vi "9870 Interface DMA (FPGA).vi"() -> ()   [LabVIEW 2014]
uses:
  <vilib>/LabVIEW Targets/FPGA/cRIO/shared/nicrio_ModuleControls/nicrio_cRIO-9871_BaudRateEnum.ctl
  <vilib>/LabVIEW Targets/FPGA/cRIO/shared/nicrio_ModuleControls/nicrio_cRIO-9871_DataBitsEnum.ctl
  <vilib>/LabVIEW Targets/FPGA/cRIO/shared/nicrio_ModuleControls/nicrio_cRIO-9871_ParityEnum.ctl
  <vilib>/LabVIEW Targets/FPGA/cRIO/shared/nicrio_ModuleControls/nicrio_cRIO-9871_StopBitsEnum.ctl
  <vilib>/LabVIEW Targets/FPGA/cRIO/shared/nicrio_ModuleControls/nicrio_cRIO-9871_FlowControlEnum.ctl
  <vilib>/rvi/Emulation/niFpgaGetClockAttributes.vi
  <vilib>/rvi/Emulation/niFpgaSctlEmulationGetInTimedLoop.vi
  <vilib>/rvi/Emulation/niFpgaEmulationReportErrorSimple.vi
  <vilib>/rvi/Emulation/niFpgaProcessEmulError.vi
  <vilib>/rvi/interface/RandomDataEmulation/niFpgaRandomDataHandleErrors.vi
  <vilib>/rvi/eio/common/nirviEmuTemplateMethod_errors.vi
  <vilib>/rvi/Emulation/niFpgaCriticalErrorInLSC.vi
  <vilib>/rvi/eio/common/nirviEmuTemplatePropertySet_errors.vi
  <vilib>/rvi/DataTransferAndStorage/Container/XNode/niFpgaContainer.xnode
  <vilib>/rvi/interface/RandomDataEmulation/nirviRandomDataFpgaReadWriteTemplate.vi
  <vilib>/eio/EIOMethodNode/EIOMethodNode.xnode
  <vilib>/eio/EIOPropertyNode/EIOPropertyNode.xnode
  <vilib>/rvi/eio/common/nirviEmuTemplatePropertyGet_errors.vi
  <vilib>/rvi/eio/common/nirviEmuTemplatePropertyGet_noerrors.vi
  <vilib>/rvi/eio/common/nirviEmuTemplatePropertySet_noerrors.vi
panel:
  in  "Write Data (FPGA2)":bool
  in  "Bytes to Send 2":i32
  in  "Port To Write (FPGA2)":enum8{"0", "1", "2", "3", "4"}(ring)
  out "error out 4b":errorcluster
  in  "Port 8":T6={"Baud Rate"=enum."9600 bps", "Data Bits"=enum."8", "Parity"=enum."None", "Stop Bits"=enum."1", "Flow Control"=enum."None"}
  in  "Port 7":T6={"Baud Rate"=enum."9600 bps", "Data Bits"=enum."8", "Parity"=enum."None", "Stop Bits"=enum."1", "Flow Control"=enum."None"}
  in  "Port 6":T6={"Baud Rate"=enum."9600 bps", "Data Bits"=enum."8", "Parity"=enum."None", "Stop Bits"=enum."1", "Flow Control"=enum."None"}
  in  "Port 5":T6={"Baud Rate"=enum."9600 bps", "Data Bits"=enum."8", "Parity"=enum."None", "Stop Bits"=enum."1", "Flow Control"=enum."None"}
  out "error out 5":errorcluster
  out "error out 6":errorcluster
  out "error out 7":errorcluster
  out "error out 8":errorcluster
  out "Error Out":errorcluster
  out "error out 4":errorcluster
  out "error out 3":errorcluster
  out "error out 2":errorcluster
  in  "Write Data (FPGA)":bool
  in  "Port To Write (FPGA)":enum8{"0", "1", "2", "3", "4"}(ring)
  in  "Port 1":T6={"Baud Rate"=enum."9600 bps", "Data Bits"=enum."8", "Parity"=enum."None", "Stop Bits"=enum."1", "Flow Control"=enum."None"}
  in  "Port 3":T6={"Baud Rate"=enum."9600 bps", "Data Bits"=enum."8", "Parity"=enum."None", "Stop Bits"=enum."1", "Flow Control"=enum."None"}
  in  "Port 4":T6={"Baud Rate"=enum."9600 bps", "Data Bits"=enum."8", "Parity"=enum."None", "Stop Bits"=enum."1", "Flow Control"=enum."None"}
  in  "Port 2":T6={"Baud Rate"=enum."9600 bps", "Data Bits"=enum."8", "Parity"=enum."None", "Stop Bits"=enum."1", "Flow Control"=enum."None"}
  in  "Bytes to Send":i32
  in  "Timeout (ms)":i32=1
  in  "Update Config":bool
  out "error out 1":errorcluster
  # "Port Read Timeout"
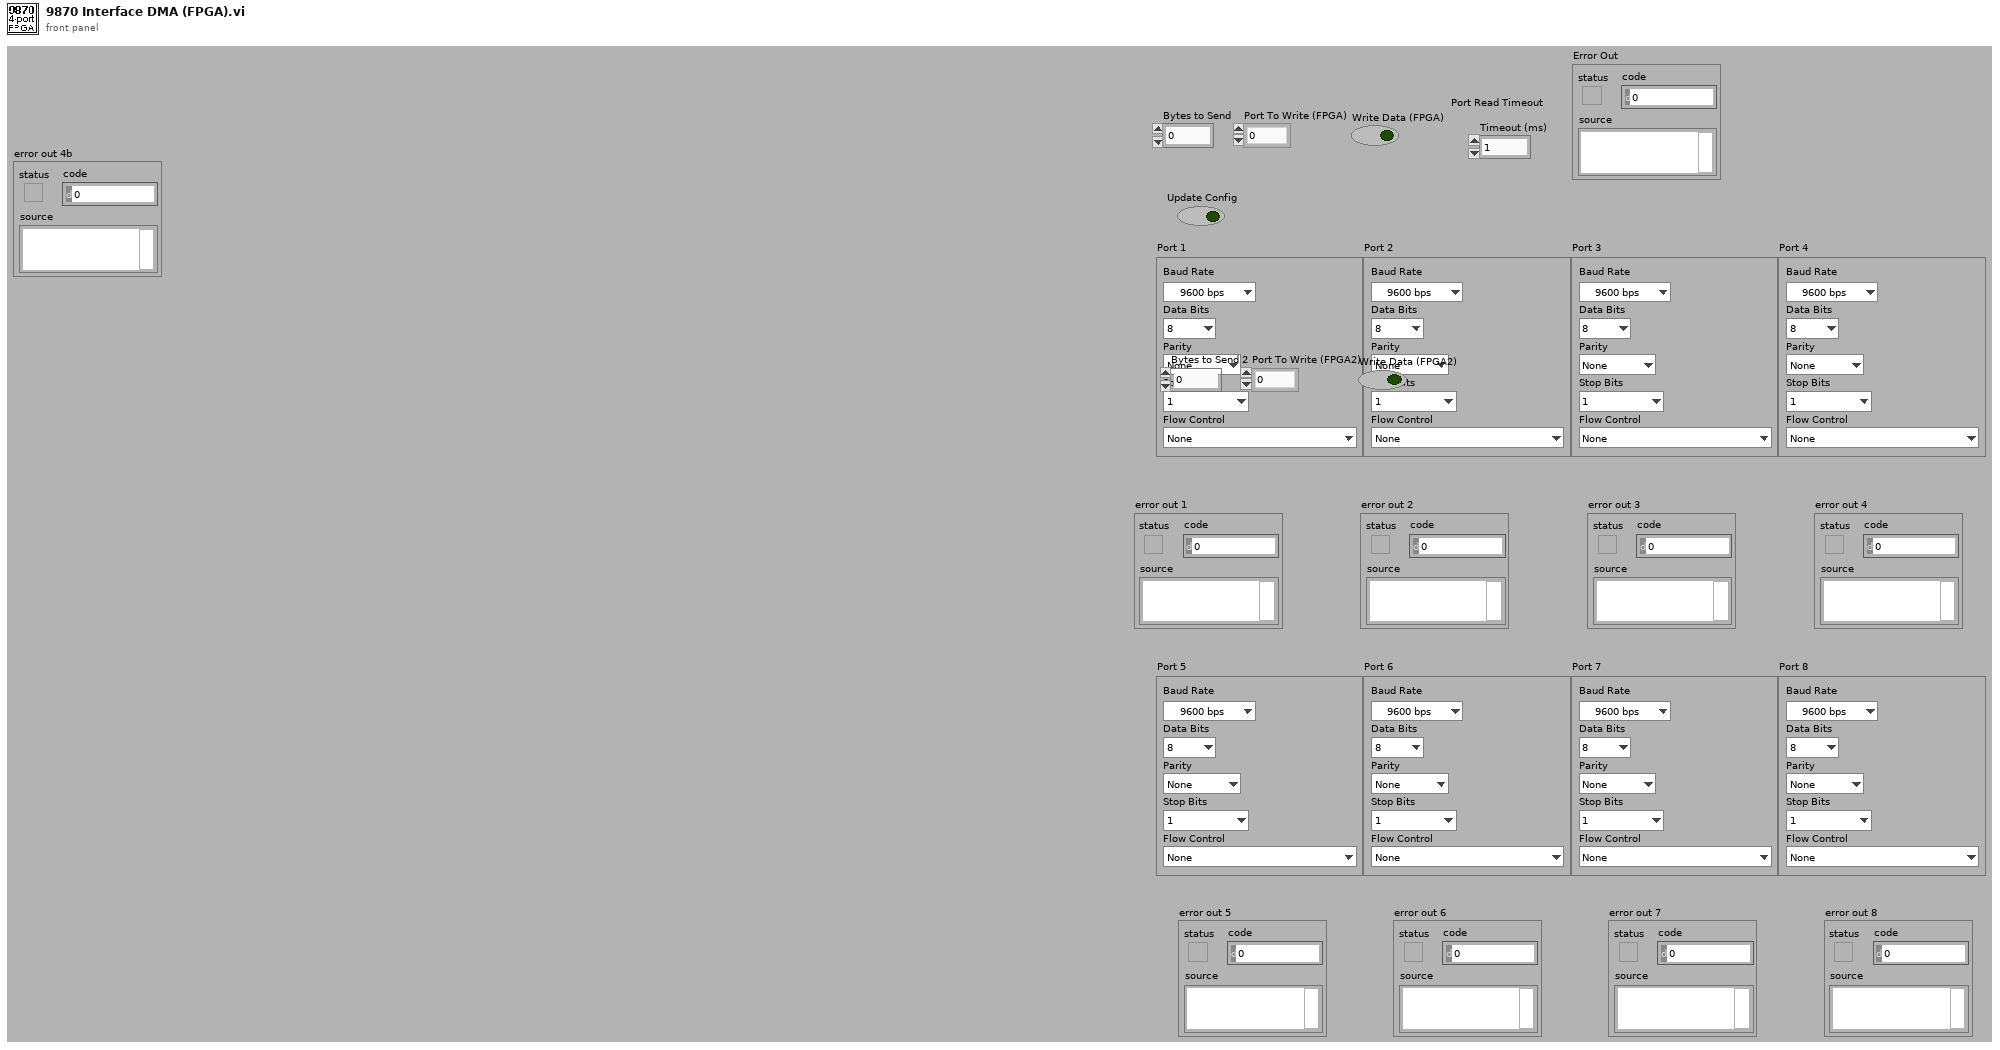
[diagram p1: front panel]
types:
  T1 = typedef "nicrio_cRIO-9871_BaudRateEnum.ctl" = enum16{"75 bps", "110 bps", "134 bps", "150 bps", "300 bps", "600 bps", "1200 bps", "1800 bps", "2400 bps", "4800 bps", "7200 bps", "9600 bps", "14.4 kbps", "19.2 kbps", "28.8 kbps", "38.4 kbps", "57.6 kbps", "115.2 kbps", "230.4 kbps", "460.8 kbps", "921.6 kbps"}
  T2 = typedef "nicrio_cRIO-9871_DataBitsEnum.ctl" = enum8{"5", "6", "7", "8"}
  T3 = typedef "nicrio_cRIO-9871_ParityEnum.ctl" = enum8{"None", "Odd", "Even", "Mark", "Space"}
  T4 = typedef "nicrio_cRIO-9871_StopBitsEnum.ctl" = enum8{"1", "1.5", "2"}
  T5 = typedef "nicrio_cRIO-9871_FlowControlEnum.ctl" = enum8{"None", "Software (XON / XOFF)", "Hardware (RTS / CTS)"}
  T6 = cluster{"Baud Rate":T1, "Data Bits":T2, "Parity":T3, "Stop Bits":T4, "Flow Control":T5}
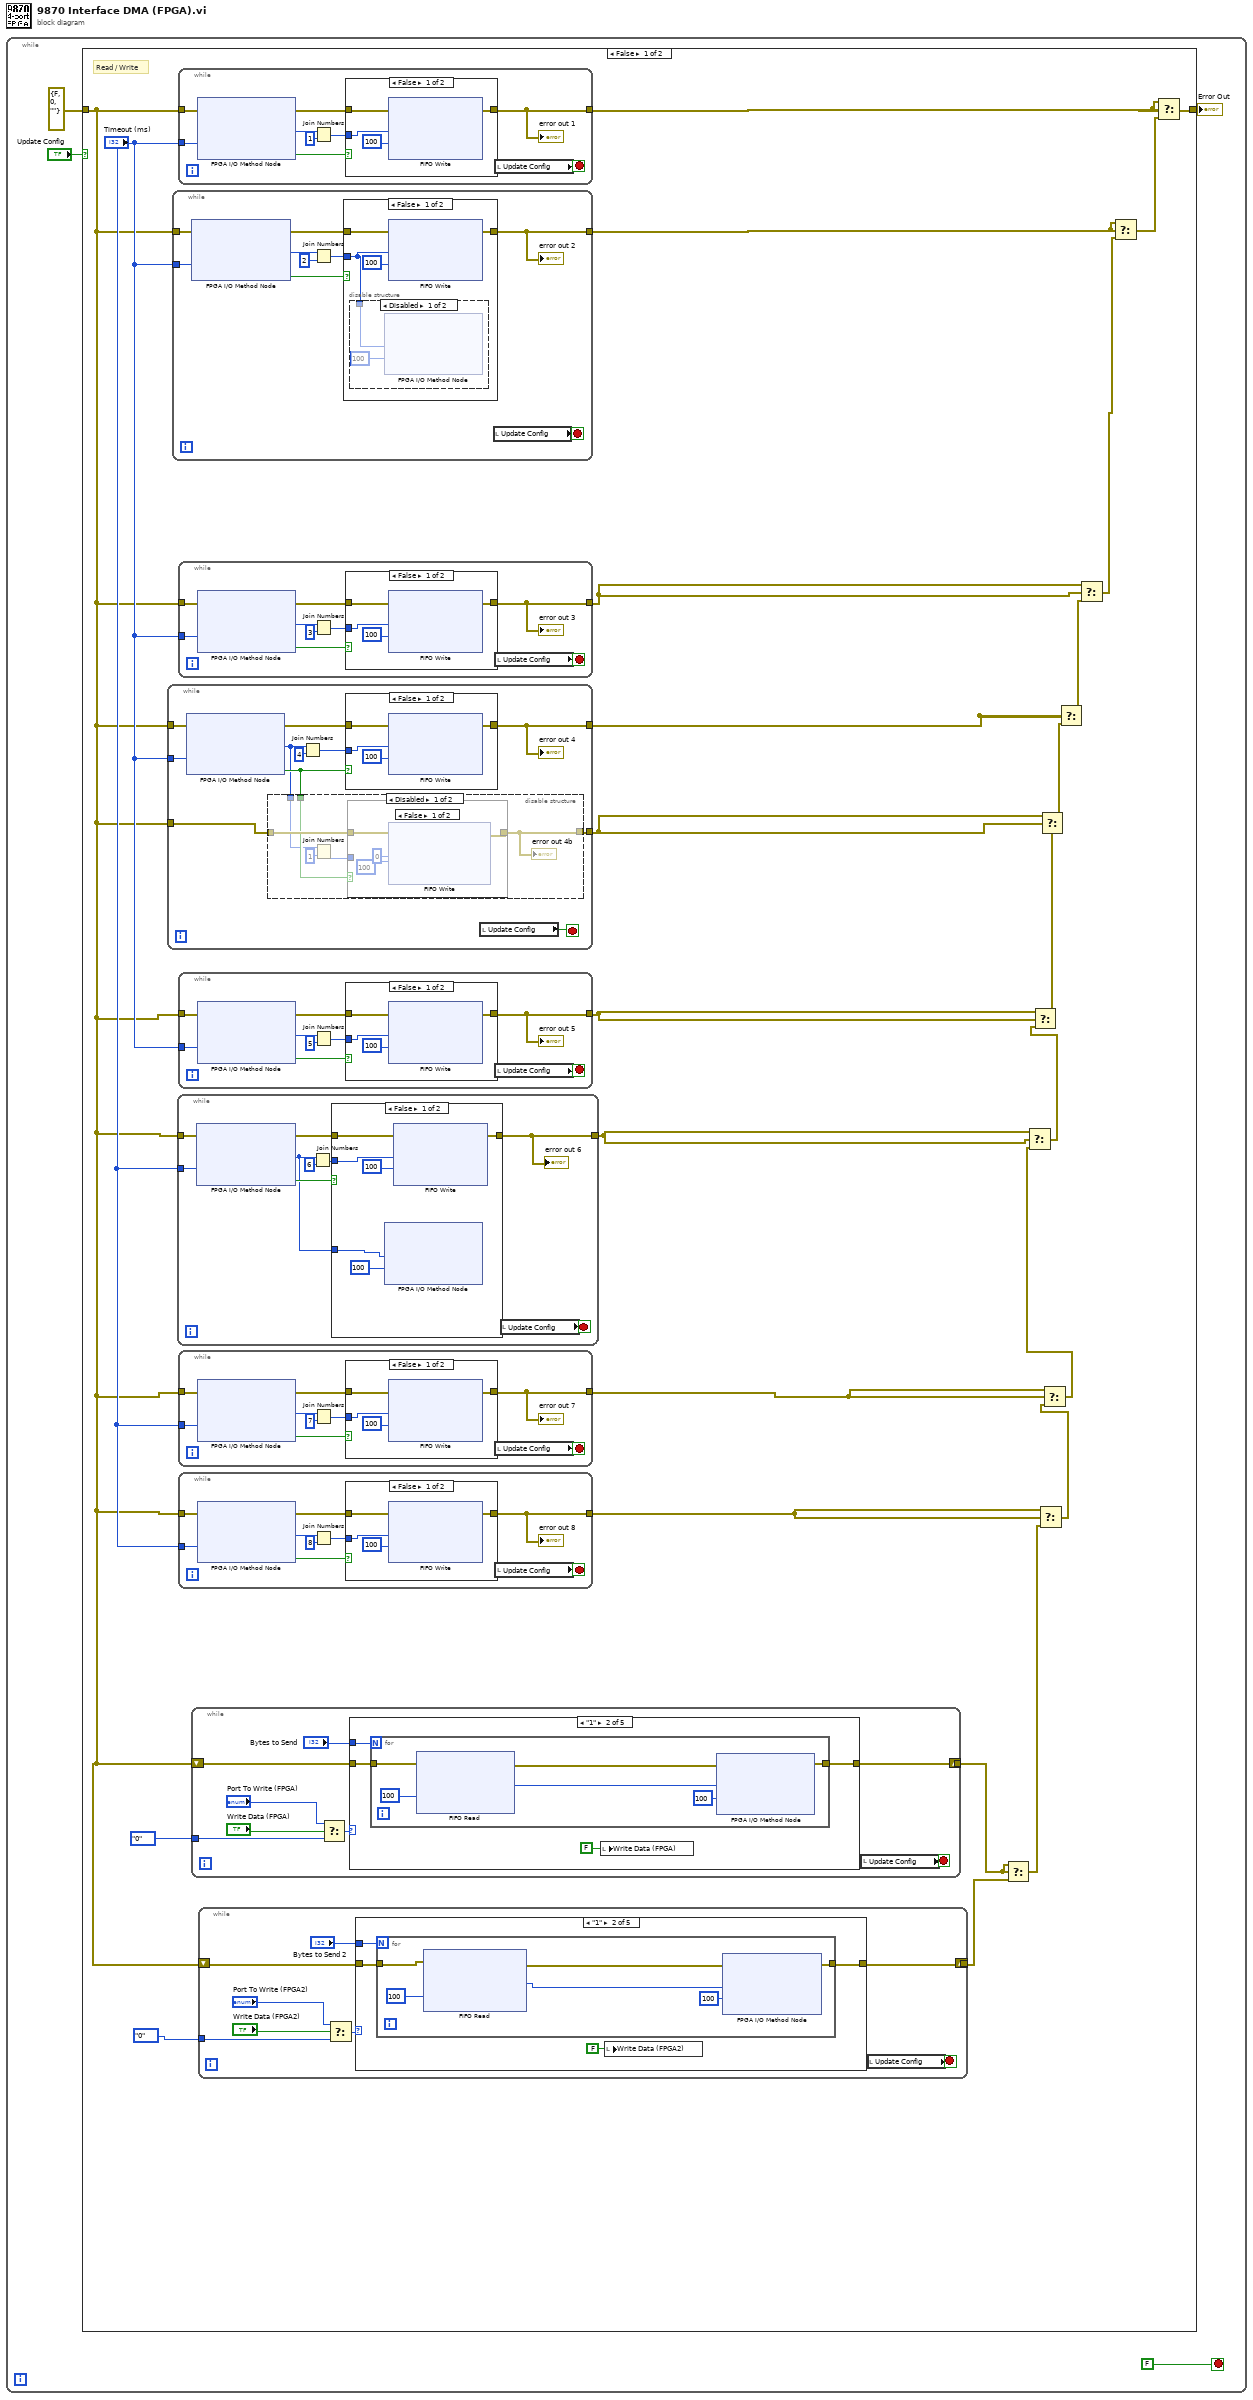
[diagram p0: block diagram]
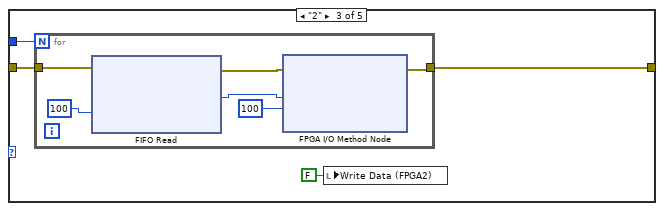
[diagram p3: hidden frame]
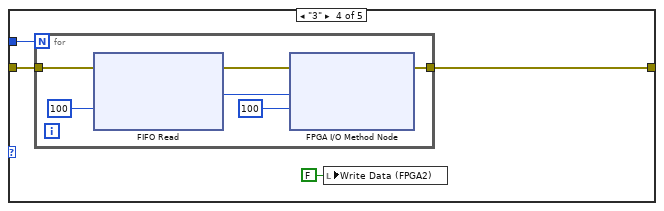
[diagram p4: hidden frame]
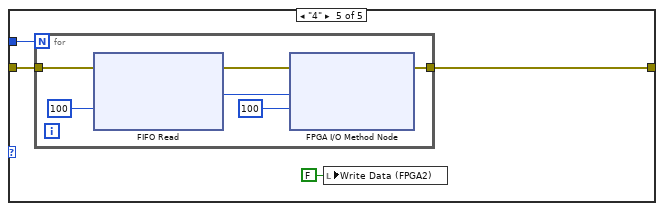
[diagram p5: hidden frame]
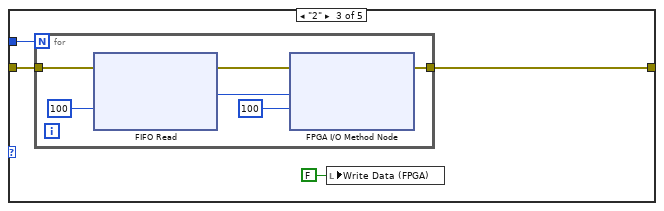
[diagram p17: hidden frame]
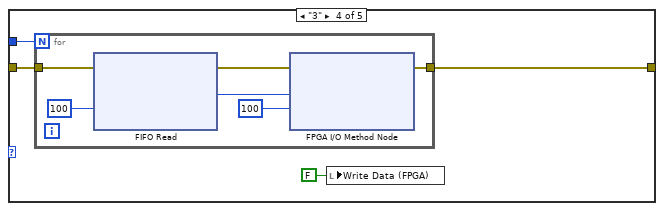
[diagram p18: hidden frame]
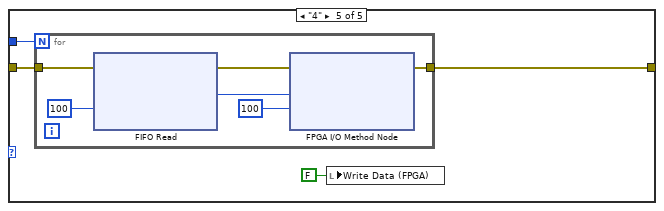
[diagram p19: hidden frame]
diagram:
  n1 = while {
    stop <- FALSE ("Boolean") stop-if-true
    n2 = case shown="False" "Update Config" {
      tunnel: [w23 w257] -> w1
      tunnel: errorcluster {"status"=FALSE, "code"=0, "source"=""} ("error out") -> [w9 w298]
      frame False {
        # "Read / Write"
        n3 = while {
          tunnel: "Timeout (ms)" -> [w144]
          tunnel: w9 -> [w147]
          tunnel: [w141] -> w22
          tunnel: w9 -> [w140]
          tunnel: [w137] -> w12
          stop <- w142 stop-if-true
          n4 = xnode "FPGA I/O Method Node"("error in"=w147, "Timeout (ms)"=w144) -> ("error out"=w143:errorcluster, "Data"=w138:u8, "Timed Out"=w139:bool)  [unwired: 1 in, 1 out]
          n5 = disable-structure shown="Disabled" {
            disable-tunnel: w140 -> [w153 _]
            disable-tunnel: w139 -> [w152 _]
            disable-tunnel: w138 -> [w151 _]
            disable-tunnel: [w150 _] -> w137
            frame Disabled {
              n6 = Join Numbers(hi=w151, lo=u8 1) -> ((hi.lo)=w148:u16)
              n7 = case shown="False" w152 {
                tunnel: w148 -> [_ _]
                tunnel: w153 -> [w157 w158]
                tunnel: [w156 w158] -> w150
                frame False {
                  n8 = xnode ("FIFO Write")("Element"=i16 0, "Timeout"=100, "error in (no error)"=w157) -> ("error out"=w156:errorcluster)  [unwired: 1 in, 2 out]
                }
                frame True {
                }
              }
              "error out 4b" <- w150
            }
            frame Enabled {
            }
          }
          n9 = Join Numbers(hi=w138, lo=u8 4) -> ((hi.lo)=w145:u16)
          n10 = case shown="False" w139 {
            tunnel: w145 -> [w161 _]
            tunnel: w143 -> [w160 w163]
            tunnel: [w159 w163] -> w141
            frame False {
              n11 = xnode ("FIFO Write")("Element"=w161, "Timeout"=100, "error in (no error)"=w160) -> ("error out"=w159:errorcluster)  [unwired: 1 in, 2 out]
            }
            frame True {
            }
          }
          "error out 4" <- w141
          n12 = local read "Update Config"() -> (w142:bool)
        }
        n13 = while {
          tunnel: "Timeout (ms)" -> [w182]
          tunnel: w9 -> [w186]
          tunnel: [w179] -> w28
          stop <- w180 stop-if-true
          n14 = xnode "FPGA I/O Method Node"("error in"=w186, "Timeout (ms)"=w182) -> ("error out"=w181:errorcluster, "Data"=w178:u8, "Timed Out"=w185:bool)  [unwired: 1 in, 1 out]
          n15 = Join Numbers(hi=w178, lo=u8 2) -> ((hi.lo)=w183:u16)
          n16 = case shown="False" w185 {
            tunnel: w183 -> [w187 _]
            tunnel: w181 -> [w189 w193]
            tunnel: [w188 w193] -> w179
            frame False {
              n17 = disable-structure shown="Disabled" {
                disable-tunnel: w187 -> [w191 _]
                frame Disabled {
                  n18 = xnode "FPGA I/O Method Node"("Data"=w191, "Timeout (ms)"=100 ("Timeout")) -> ()  [unwired: 2 in, 3 out]
                }
                frame Enabled {
                }
              }
              n19 = xnode ("FIFO Write")("Element"=w187, "Timeout"=100, "error in (no error)"=w189) -> ("error out"=w188:errorcluster)  [unwired: 1 in, 2 out]
            }
            frame True {
            }
          }
          "error out 2" <- w179
          n20 = local read "Update Config"() -> (w180:bool)
        }
        n21 = while {
          tunnel: "Timeout (ms)" -> [w111]
          tunnel: w9 -> [w115]
          tunnel: [w108] -> w15
          stop <- w109 stop-if-true
          n22 = xnode "FPGA I/O Method Node"("error in"=w115, "Timeout (ms)"=w111) -> ("error out"=w110:errorcluster, "Data"=w107:u8, "Timed Out"=w114:bool)  [unwired: 1 in, 1 out]
          n23 = Join Numbers(hi=w107, lo=u8 6) -> ((hi.lo)=w112:u16)
          n24 = case shown="False" w114 {
            tunnel: w112 -> [w120 _]
            tunnel: w110 -> [w119 w122]
            tunnel: [w118 w122] -> w108
            tunnel: w107 -> [w116 _]
            frame False {
              n25 = xnode "FPGA I/O Method Node"("Data"=w116, "Timeout (ms)"=100 ("Timeout")) -> ()  [unwired: 2 in, 3 out]
              n26 = xnode ("FIFO Write")("Element"=w120, "Timeout"=100, "error in (no error)"=w119) -> ("error out"=w118:errorcluster)  [unwired: 1 in, 2 out]
            }
            frame True {
            }
          }
          "error out 6" <- w108
          n27 = local read "Update Config"() -> (w109:bool)
        }
        n28 = while {
          tunnel: "Timeout (ms)" -> [w246]
          tunnel: w9 -> [w251]
          tunnel: [w243] -> w27
          stop <- w244 stop-if-true
          n29 = xnode "FPGA I/O Method Node"("error in"=w251, "Timeout (ms)"=w246) -> ("error out"=w245:errorcluster, "Data"=w249:u8, "Timed Out"=w250:bool)  [unwired: 1 in, 1 out]
          n30 = Join Numbers(hi=w249, lo=u8 1) -> ((hi.lo)=w247:u16)
          n31 = case shown="False" w250 {
            tunnel: w247 -> [w254 _]
            tunnel: w245 -> [w253 w256]
            tunnel: [w252 w256] -> w243
            frame False {
              n32 = xnode ("FIFO Write")("Element"=w254, "Timeout"=100, "error in (no error)"=w253) -> ("error out"=w252:errorcluster)  [unwired: 1 in, 2 out]
            }
            frame True {
            }
          }
          "error out 1" <- w243
          n33 = local read "Update Config"() -> (w244:bool)
        }
        n34 = while {
          tunnel: "Timeout (ms)" -> [w167]
          tunnel: w9 -> [w172]
          tunnel: [w164] -> w26
          stop <- w165 stop-if-true
          n35 = xnode "FPGA I/O Method Node"("error in"=w172, "Timeout (ms)"=w167) -> ("error out"=w166:errorcluster, "Data"=w170:u8, "Timed Out"=w171:bool)  [unwired: 1 in, 1 out]
          n36 = Join Numbers(hi=w170, lo=u8 3) -> ((hi.lo)=w168:u16)
          n37 = case shown="False" w171 {
            tunnel: w168 -> [w175 _]
            tunnel: w166 -> [w174 w177]
            tunnel: [w173 w177] -> w164
            frame False {
              n38 = xnode ("FIFO Write")("Element"=w175, "Timeout"=100, "error in (no error)"=w174) -> ("error out"=w173:errorcluster)  [unwired: 1 in, 2 out]
            }
            frame True {
            }
          }
          "error out 3" <- w164
          n39 = local read "Update Config"() -> (w165:bool)
        }
        n40 = while {
          tunnel: "Timeout (ms)" -> [w126]
          tunnel: w9 -> [w131]
          tunnel: [w123] -> w16
          stop <- w124 stop-if-true
          n41 = xnode "FPGA I/O Method Node"("error in"=w131, "Timeout (ms)"=w126) -> ("error out"=w125:errorcluster, "Data"=w129:u8, "Timed Out"=w130:bool)  [unwired: 1 in, 1 out]
          n42 = Join Numbers(hi=w129, lo=u8 5) -> ((hi.lo)=w127:u16)
          n43 = case shown="False" w130 {
            tunnel: w127 -> [w134 _]
            tunnel: w125 -> [w133 w136]
            tunnel: [w132 w136] -> w123
            frame False {
              n44 = xnode ("FIFO Write")("Element"=w134, "Timeout"=100, "error in (no error)"=w133) -> ("error out"=w132:errorcluster)  [unwired: 1 in, 2 out]
            }
            frame True {
            }
          }
          "error out 5" <- w123
          n45 = local read "Update Config"() -> (w124:bool)
        }
        n46 = while {
          tunnel: "Timeout (ms)" -> [w96]
          tunnel: w9 -> [w101]
          tunnel: [w93] -> w14
          stop <- w94 stop-if-true
          n47 = xnode "FPGA I/O Method Node"("error in"=w101, "Timeout (ms)"=w96) -> ("error out"=w95:errorcluster, "Data"=w99:u8, "Timed Out"=w100:bool)  [unwired: 1 in, 1 out]
          n48 = Join Numbers(hi=w99, lo=u8 7) -> ((hi.lo)=w97:u16)
          n49 = case shown="False" w100 {
            tunnel: w97 -> [w104 _]
            tunnel: w95 -> [w103 w106]
            tunnel: [w102 w106] -> w93
            frame False {
              n50 = xnode ("FIFO Write")("Element"=w104, "Timeout"=100, "error in (no error)"=w103) -> ("error out"=w102:errorcluster)  [unwired: 1 in, 2 out]
            }
            frame True {
            }
          }
          "error out 7" <- w93
          n51 = local read "Update Config"() -> (w94:bool)
        }
        n52 = while {
          tunnel: "Timeout (ms)" -> [w82]
          tunnel: w9 -> [w87]
          tunnel: [w79] -> w13
          stop <- w80 stop-if-true
          n53 = xnode "FPGA I/O Method Node"("error in"=w87, "Timeout (ms)"=w82) -> ("error out"=w81:errorcluster, "Data"=w85:u8, "Timed Out"=w86:bool)  [unwired: 1 in, 1 out]
          n54 = Join Numbers(hi=w85, lo=u8 8) -> ((hi.lo)=w83:u16)
          n55 = case shown="False" w86 {
            tunnel: w83 -> [w90 _]
            tunnel: w81 -> [w89 w92]
            tunnel: [w88 w92] -> w79
            frame False {
              n56 = xnode ("FIFO Write")("Element"=w90, "Timeout"=100, "error in (no error)"=w89) -> ("error out"=w88:errorcluster)  [unwired: 1 in, 2 out]
            }
            frame True {
            }
          }
          "error out 8" <- w79
          n57 = local read "Update Config"() -> (w80:bool)
        }
        n58 = while {
          shift-right: [w198] -> _
          shift-left: w9 -> [w201]
          tunnel: enum8{"0", "1", "2", "3", "4"}."0" ("Port To Write (FPGA) 2") -> [w196]
          tunnel: [w198] -> w6
          stop <- w200 stop-if-true
          n59 = Select(t="Port To Write (FPGA)", s="Write Data (FPGA)", f=w196) -> (s? t:f=w195:enum8{"0", "1", "2", "3", "4"})
          n60 = case shown="\"1\"" w195 {
            tunnel: w201 -> [w202 w206 w216 w226 w236]
            tunnel: "Bytes to Send" -> [_ w205 w215 w225 w235]
            tunnel: [w202 w204 w214 w224 w234] -> w198
            frame "0", Default {
            }
            frame "1" {
              n61 = for {
                N: w205 -> [_]
                tunnel: w206 -> [w212]
                tunnel: [w208] -> w204
                n62 = xnode ("FIFO Read")("Timeout"=100 ("Timeout (ms)"), "error in (no error)"=w212) -> ("Element"=w207:u8, "error out"=w211:errorcluster)  [unwired: 1 in, 2 out]
                n63 = xnode "FPGA I/O Method Node"("error in"=w211, "Data"=w207, "Timeout (ms)"=100) -> ("error out"=w208:errorcluster)  [unwired: 1 in, 2 out]
              }
              n64 = local write "Write Data (FPGA)"(FALSE ("Write Data (FPGA)")) -> ()
            }
            frame "2" {
              n65 = for {
                N: w215 -> [_]
                tunnel: w216 -> [w221]
                tunnel: [w217] -> w214
                n66 = xnode ("FIFO Read")("Timeout"=100 ("Timeout (ms)"), "error in (no error)"=w221) -> ("Element"=w222:u8, "error out"=w220:errorcluster)  [unwired: 1 in, 2 out]
                n67 = xnode "FPGA I/O Method Node"("error in"=w220, "Data"=w222, "Timeout (ms)"=100) -> ("error out"=w217:errorcluster)  [unwired: 1 in, 2 out]
              }
              n68 = local write "Write Data (FPGA)"(FALSE ("Write Data (FPGA)")) -> ()
            }
            frame "3" {
              n69 = for {
                N: w225 -> [_]
                tunnel: w226 -> [w231]
                tunnel: [w227] -> w224
                n70 = xnode ("FIFO Read")("Timeout"=100 ("Timeout (ms)"), "error in (no error)"=w231) -> ("Element"=w232:u8, "error out"=w230:errorcluster)  [unwired: 1 in, 2 out]
                n71 = xnode "FPGA I/O Method Node"("error in"=w230, "Data"=w232, "Timeout (ms)"=100) -> ("error out"=w227:errorcluster)  [unwired: 1 in, 2 out]
              }
              n72 = local write "Write Data (FPGA)"(FALSE ("Write Data (FPGA)")) -> ()
            }
            frame "4" {
              n73 = for {
                N: w235 -> [_]
                tunnel: w236 -> [w241]
                tunnel: [w237] -> w234
                n74 = xnode ("FIFO Read")("Timeout"=100 ("Timeout (ms)"), "error in (no error)"=w241) -> ("Element"=w242:u8, "error out"=w240:errorcluster)  [unwired: 1 in, 2 out]
                n75 = xnode "FPGA I/O Method Node"("error in"=w240, "Data"=w242, "Timeout (ms)"=100) -> ("error out"=w237:errorcluster)  [unwired: 1 in, 2 out]
              }
              n76 = local write "Write Data (FPGA)"(FALSE ("Write Data (FPGA)")) -> ()
            }
          }
          n77 = local read "Update Config"() -> (w200:bool)
        }
        n78 = while {
          shift-right: [w34] -> w7
          shift-left: w9 -> [w37]
          tunnel: enum8{"0", "1", "2", "3", "4"}."0" ("Port To Write (FPGA) 2") -> [w32]
          tunnel: [w34] -> _
          stop <- w36 stop-if-true
          n79 = Select(t="Port To Write (FPGA2)", s="Write Data (FPGA2)", f=w32) -> (s? t:f=w31:enum8{"0", "1", "2", "3", "4"})
          n80 = case shown="\"1\"" w31 {
            tunnel: w37 -> [w38 w42 w52 w62 w72]
            tunnel: "Bytes to Send 2" -> [_ w41 w51 w61 w71]
            tunnel: [w38 w40 w50 w60 w70] -> w34
            frame "0", Default {
            }
            frame "1" {
              n81 = for {
                N: w41 -> [_]
                tunnel: w42 -> [w48]
                tunnel: [w45] -> w40
                n82 = xnode ("FIFO Read")("Timeout"=100 ("Timeout (ms)"), "error in (no error)"=w48) -> ("Element"=w43:i16, "error out"=w47:errorcluster)  [unwired: 1 in, 2 out]
                n83 = xnode "FPGA I/O Method Node"("error in"=w47, "Data"=w43, "Timeout (ms)"=100) -> ("error out"=w45:errorcluster)  [unwired: 1 in, 2 out]
              }
              n84 = local write "Write Data (FPGA2)"(FALSE ("Write Data (FPGA)")) -> ()
            }
            frame "2" {
              n85 = for {
                N: w51 -> [_]
                tunnel: w52 -> [w58]
                tunnel: [w53] -> w50
                n86 = xnode ("FIFO Read")("Timeout"=100 ("Timeout (ms)"), "error in (no error)"=w58) -> ("Element"=w56:i16, "error out"=w54:errorcluster)  [unwired: 1 in, 2 out]
                n87 = xnode "FPGA I/O Method Node"("error in"=w54, "Data"=w56, "Timeout (ms)"=100) -> ("error out"=w53:errorcluster)  [unwired: 1 in, 2 out]
              }
              n88 = local write "Write Data (FPGA2)"(FALSE ("Write Data (FPGA)")) -> ()
            }
            frame "3" {
              n89 = for {
                N: w61 -> [_]
                tunnel: w62 -> [w67]
                tunnel: [w63] -> w60
                n90 = xnode ("FIFO Read")("Timeout"=100 ("Timeout (ms)"), "error in (no error)"=w67) -> ("Element"=w68:i16, "error out"=w66:errorcluster)  [unwired: 1 in, 2 out]
                n91 = xnode "FPGA I/O Method Node"("error in"=w66, "Data"=w68, "Timeout (ms)"=100) -> ("error out"=w63:errorcluster)  [unwired: 1 in, 2 out]
              }
              n92 = local write "Write Data (FPGA2)"(FALSE ("Write Data (FPGA)")) -> ()
            }
            frame "4" {
              n93 = for {
                N: w71 -> [_]
                tunnel: w72 -> [w77]
                tunnel: [w73] -> w70
                n94 = xnode ("FIFO Read")("Timeout"=100 ("Timeout (ms)"), "error in (no error)"=w77) -> ("Element"=w78:i16, "error out"=w76:errorcluster)  [unwired: 1 in, 2 out]
                n95 = xnode "FPGA I/O Method Node"("error in"=w76, "Data"=w78, "Timeout (ms)"=100) -> ("error out"=w73:errorcluster)  [unwired: 1 in, 2 out]
              }
              n96 = local write "Write Data (FPGA2)"(FALSE ("Write Data (FPGA)")) -> ()
            }
          }
          n97 = local read "Update Config"() -> (w36:bool)
        }
        n98 = Select(t=w6, s=w6, f=w7) -> (s? t:f=w5:errorcluster)
        n99 = Select(t=w13, s=w13, f=w5) -> (s? t:f=w17:errorcluster)
        n100 = Select(t=w14, s=w14, f=w17) -> (s? t:f=w18:errorcluster)
        n101 = Select(t=w15, s=w15, f=w18) -> (s? t:f=w19:errorcluster)
        n102 = Select(t=w16, s=w16, f=w19) -> (s? t:f=w11:errorcluster)
        n103 = Select(t=w12, s=w12, f=w11) -> (s? t:f=w10:errorcluster)
        n104 = Select(t=w22, s=w22, f=w10) -> (s? t:f=w21:errorcluster)
        n105 = Select(t=w26, s=w26, f=w21) -> (s? t:f=w24:errorcluster)
        n106 = Select(t=w28, s=w28, f=w24) -> (s? t:f=w25:errorcluster)
        n107 = Select(t=w27, s=w27, f=w25) -> (s? t:f=w23:errorcluster)
      }
      frame True {
        # "UPDATE Configuration"
        n108 = Unbundle By Name("Port 1") -> ("Baud Rate"=w321:T1, "Data Bits"=w320:T2, "Parity"=w319:T3, "Stop Bits"=w318:T4, "Flow Control"=w317:T5)
        n109 = Unbundle By Name("Port 3") -> ("Baud Rate"=w305:T1, "Data Bits"=w306:T2, "Parity"=w307:T3, "Stop Bits"=w308:T4, "Flow Control"=w309:T5)
        n110 = Unbundle By Name("Port 5") -> ("Baud Rate"=w269:T1, "Data Bits"=w270:T2, "Parity"=w271:T3, "Stop Bits"=w272:T4, "Flow Control"=w273:T5)
        n111 = Unbundle By Name("Port 7") -> ("Baud Rate"=w279:T1, "Data Bits"=w278:T2, "Parity"=w277:T3, "Stop Bits"=w276:T4, "Flow Control"=w275:T5)
        n112 = xnode "FPGA I/O Property Node"("error in"=w298, "Baud Rate"=w321, "Data Bits"=w320, "Parity"=w319, "Stop Bits"=w318, "Flow Control"=w317) -> ("error out"=w296:errorcluster)  [unwired: 1 in, 1 out]
        n113 = xnode "FPGA I/O Method Node"("error in"=w296) -> ("error out"=w295:errorcluster)  [unwired: 1 in, 1 out]
        n114 = Unbundle By Name("Port 2") -> ("Baud Rate"=w315:T1, "Data Bits"=w314:T2, "Parity"=w313:T3, "Stop Bits"=w312:T4, "Flow Control"=w311:T5)
        n115 = Unbundle By Name("Port 4") -> ("Baud Rate"=w299:T1, "Data Bits"=w300:T2, "Parity"=w301:T3, "Stop Bits"=w302:T4, "Flow Control"=w303:T5)
        n116 = Unbundle By Name("Port 6") -> ("Baud Rate"=w285:T1, "Data Bits"=w284:T2, "Parity"=w283:T3, "Stop Bits"=w282:T4, "Flow Control"=w281:T5)
        n117 = Unbundle By Name("Port 8") -> ("Baud Rate"=w263:T1, "Data Bits"=w264:T2, "Parity"=w265:T3, "Stop Bits"=w266:T4, "Flow Control"=w267:T5)
        n118 = xnode "FPGA I/O Property Node"("error in"=w295, "Baud Rate"=w315, "Data Bits"=w314, "Parity"=w313, "Stop Bits"=w312, "Flow Control"=w311) -> ("error out"=w294:errorcluster)  [unwired: 1 in, 1 out]
        n119 = xnode "FPGA I/O Method Node"("error in"=w294) -> ("error out"=w293:errorcluster)  [unwired: 1 in, 1 out]
        n120 = xnode "FPGA I/O Property Node"("error in"=w293, "Baud Rate"=w305, "Data Bits"=w306, "Parity"=w307, "Stop Bits"=w308, "Flow Control"=w309) -> ("error out"=w292:errorcluster)  [unwired: 1 in, 1 out]
        n121 = xnode "FPGA I/O Method Node"("error in"=w292) -> ("error out"=w291:errorcluster)  [unwired: 1 in, 1 out]
        n122 = xnode "FPGA I/O Property Node"("error in"=w291, "Baud Rate"=w299, "Data Bits"=w300, "Parity"=w301, "Stop Bits"=w302, "Flow Control"=w303) -> ("error out"=w290:errorcluster)  [unwired: 1 in, 1 out]
        n123 = xnode "FPGA I/O Method Node"("error in"=w290) -> ("error out"=w261:errorcluster)  [unwired: 1 in, 1 out]
        n124 = xnode "FPGA I/O Property Node"("error in"=w261, "Baud Rate"=w269, "Data Bits"=w270, "Parity"=w271, "Stop Bits"=w272, "Flow Control"=w273) -> ("error out"=w287:errorcluster)  [unwired: 1 in, 1 out]
        n125 = xnode "FPGA I/O Method Node"("error in"=w287) -> ("error out"=w260:errorcluster)  [unwired: 1 in, 1 out]
        n126 = xnode "FPGA I/O Property Node"("error in"=w260, "Baud Rate"=w285, "Data Bits"=w284, "Parity"=w283, "Stop Bits"=w282, "Flow Control"=w281) -> ("error out"=w289:errorcluster)  [unwired: 1 in, 1 out]
        n127 = xnode "FPGA I/O Method Node"("error in"=w289) -> ("error out"=w259:errorcluster)  [unwired: 1 in, 1 out]
        n128 = xnode "FPGA I/O Property Node"("error in"=w259, "Baud Rate"=w279, "Data Bits"=w278, "Parity"=w277, "Stop Bits"=w276, "Flow Control"=w275) -> ("error out"=w288:errorcluster)  [unwired: 1 in, 1 out]
        n129 = xnode "FPGA I/O Method Node"("error in"=w288) -> ("error out"=w258:errorcluster)  [unwired: 1 in, 1 out]
        n130 = xnode "FPGA I/O Property Node"("error in"=w258, "Baud Rate"=w263, "Data Bits"=w264, "Parity"=w265, "Stop Bits"=w266, "Flow Control"=w267) -> ("error out"=w286:errorcluster)  [unwired: 1 in, 1 out]
        n131 = xnode "FPGA I/O Method Node"("error in"=w286) -> ("error out"=w257:errorcluster)  [unwired: 1 in, 1 out]
        n132 = local write "Update Config"(FALSE ("Update Config")) -> ()
      }
    }
    "Error Out" <- w1
  }
